vi "ReadAvi.vi"() -> ()   [LabVIEW 2015]
panel:
  out "Image":T1(plugin-control)
  in  "Stop":bool
  out "Progress Bar":i32(slide) max=115 scale=1.0..115.0
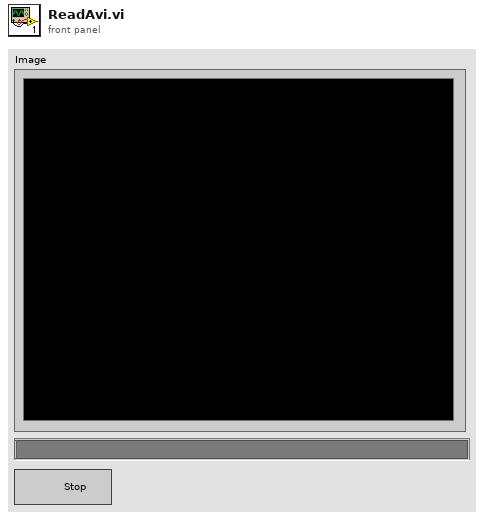
[diagram p1: front panel]
types:
  T1 = typedef "IMAQ Image.ctl" = refnum<image>
  T2 = typedef "IMAQ AVI2 Refnum.ctl" = refnum<k20>
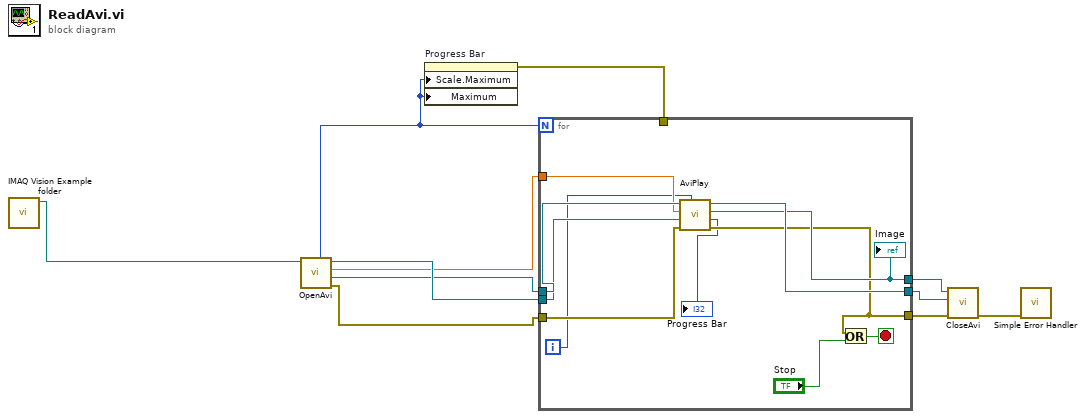
[diagram p0: block diagram]
diagram:
  n1 = call "IMAQ Vision Example folder.vi"() -> ("Example Image Path"=w3:path)  [unwired: 11 in]
  n2 = call "OpenAvi.vi"("Example Image Path"=w3) -> ("error out"=w8:errorcluster, "AVI Refnum (duplicate)"=w6:T2, "Numeric"=w4:dbl, "Refnum out"=w7:T1, "Number of Frames"=w2:u32)  [unwired: 6 in]
  n3 = property on="Progress Bar" class="Slide (strict)"("Scale.Maximum"=w2, "Maximum"=w2) -> (error out=w1:errorcluster)  [unwired: 2 in, 1 out]
  n4 = for {
    N: w2 -> [_]
    tunnel: w7 -> [w21]
    tunnel: [w20] -> w9
    tunnel: [w16] -> w10
    tunnel: w8 -> [w19]
    tunnel: w6 -> [w22]
    tunnel: [w17] -> w5
    tunnel: w4 -> [w18]
    tunnel: w1 -> [_]
    i -> [w13]
    stop <- w14 stop-if-true
    n5 = call "AviPlay.vi"("Numeric"=w13, "error in (no error)"=w19, "New Image"=w21, "Seconds per Frame"=w18, "Refnum in"=w22) -> ("error out"=w16:errorcluster, "Progress Bar"=→"Progress Bar":i32, "Image Out"=w17:T1, "Refnum out"=w20:T2)  [unwired: 3 in]
    "Image" <- w17
    n6 = Or(x=w16, y="Stop") -> (x .or. y?=w14:bool)
  }
  n7 = call "CloseAvi.vi"("error in (no error)"=w10, 10:"Refnum in"=w9, 11:"Refnum in"=w5) -> ("error out"=w11:errorcluster)  [unwired: 8 in]
  n8 = call <vilib>:"Simple Error Handler.vi"("error in (no error)"=w11) -> ()  [unwired: 1 in, 8 out]
